vi "Func2.vi"   [LabVIEW 2014, in "Plugin Template.lvlib"]
uses:
  Plugin Template.lvlib
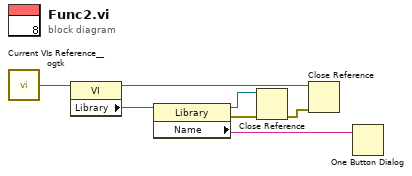
[diagram p0: block diagram]
diagram:
  n1 = call <userlib>:"Current VIs Reference__ogtk.vi"() -> ("Current VI's reference"=w7:refnum<vi>)  [unwired: 5 in]
  n2 = property class="VI"(reference=w7) -> (reference out=w1:refnum<vi>, "Library"=w6:refnum<vi>)  [unwired: 1 in, 1 out]
  n3 = property class="Library"(reference=w6) -> (reference out=w3:refnum<vi>, error out=w4:errorcluster, "Name"=w5:string)  [unwired: 1 in]
  n4 = Close Reference(reference=w3, error in (no error)=w4) -> (error out=w2:errorcluster)
  n5 = Close Reference(reference=w1, error in (no error)=w2) -> ()  [unwired: 1 out]
  n6 = One Button Dialog(message=w5) -> ()  [unwired: 1 in, 1 out]
